vi "Pre Launch Init.vi"(11 "Template in":refnum<class "Template.lvclass">) -> (0 "error out":errorcluster, 3 "Template out":refnum<class "Template.lvclass">)   [LabVIEW 2020, in "Template.lvlib" / "Template.lvclass"]
doc: "(<B>Filename</B>: Actor Framework.lvlib:Actor.lvclass:Pre Launch Init.vi)\n\nDefines behavior that occurs after the Launch Nested Actor method is invoked but before the actor's Actor Core method begins running.\n\nBy default, this method does nothing. A descendant class may override it to define behavior."
uses:
  Template.lvclass
  Template.lvclass/Template.ctl
  <vilib>/ActorFramework/Actor/Actor.lvclass
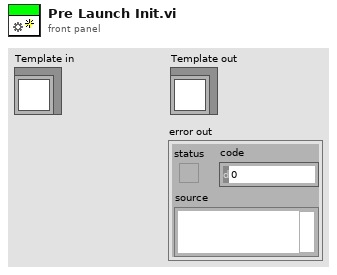
[diagram p1: front panel]
types:
  T1 = typedef "Template.lvlib/Template.lvclass/actor configuration.ctl" = cluster{"GlobalConfiguration":T2, "DeviceConfiguration":T3}
  T2 = typedef "Template.lvlib/Template.lvclass/shared actor configuration.ctl" = cluster{"DeviceFamily":string, "WriteData":bool, "BufferSize":i32, "SyncDevice":bool, "ExecuteInterruptRoutine":bool, "InterruptRoutineTimeout":i32}
  T3 = typedef "Template.lvlib/Template.lvclass/device configuration cluster.ctl" = cluster{"DeviceSpecificName":string, "HardwareReference":string, "UsedResources":T4[]}
  T4 = typedef "Template.lvlib/Template.lvclass/single resource cluster.ctl" = cluster{"ResourceLocation":string, "ResourceData":variant}
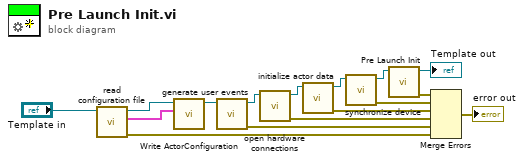
[diagram p0: block diagram]
diagram:
  n1 = call-dynamic "read configuration file.vi"("Template in"="Template in") -> ("error out"=w3:errorcluster, "ActorConfiguration"=w1:T1, "Template out"=w10:refnum<class "Template.lvclass">)  [unwired: 8 in]
  n2 = call "Write ActorConfiguration.vi"("ActorConfiguration"=w1, "Template in"=w10) -> ("Template out"=w2:refnum<class "Template.lvclass">)  [unwired: 9 in]
  n3 = call-dynamic "generate user events.vi"("Template in"=w2) -> ("error out"=w4:errorcluster, "Template out"=w13:refnum<class "Template.lvclass">)  [unwired: 9 in]
  n4 = call-dynamic "open hardware connections.vi"("Template in"=w13) -> ("error out"=w5:errorcluster, "Template out"=w9:refnum<class "Template.lvclass">)  [unwired: 9 in]
  n5 = call-dynamic "initialize actor data.vi"("Template in"=w9) -> ("error out"=w6:errorcluster, "Template out"=w12:refnum<class "Template.lvclass">)  [unwired: 9 in]
  n6 = call-dynamic "synchronize device.vi"("Template in"=w12) -> ("error out"=w7:errorcluster, "Template out"=w8:refnum<class "Template.lvclass">)  [unwired: 9 in]
  n7 = call-parent "Pre Launch Init.vi"("Actor in"=w8) -> ("error out"=w16:errorcluster, "Actor out"=→"Template out":refnum<class "Template.lvclass">)  [unwired: 9 in]
  n8 = Merge Errors(w16, w7, w6, w5, w4, w3) -> (→"error out":errorcluster)
